vi "Get Module and FPGA Data.vi"(8 "error in (no error)":errorcluster, 11 "Parent Ref in":T2 format="%.0x") -> (0 "error out":errorcluster, 1 "RSI Modules":T10[](array[typedef]) {"Module Config Data"."Config Block Data Refs"."Data Reference" format="%.0x"; "CDOutput Data"."BD Refs"."Data Reference" format="%.0x"; "CDInput Data"."BD Refs"."Data Reference" format="%.0x"; "VS ref" format="%.0x"}, 2 "FPGA":T1[](array[typedef]) {"UDVs"."To FPGA"."VS ref" format="%.0x"; "UDVs"."From FPGA"."VS ref" format="%.0x"; "VS ref" format="%.0x"; "Output Data"."BD Refs"."Data Reference" format="%.0x"; "Input Data"."BD Refs"."Data Reference" format="%.0x"}, 3 "Parent Ref out":T2 format="%.0x", 4 "FPGALoaded":bool)   [LabVIEW 2020, in "SEECD Engine.lvlib"]
uses:
  SEECD Engine.lvlib
  <vilib>/NI VeriStand/Custom Device API/Custom Device API.lvlib
  Shared/Globals/Scan Engine GUIDs.vi
  Shared/SEECD Shared.lvlib
  <vilib>/NI VeriStand/Custom Device API/Custom Device Item Ref.ctl
  Includes/Modules.lvlibp/RSI Module/RSI Module.lvclass
  Includes/Modules.lvlibp/RSI Module/Module Models.ctl
  <vilib>/NI VeriStand/Custom Device API/Data Reference.ctl
  <vilib>/NI VeriStand/Custom Device API/Block Data Reference.ctl
  Type Defs/RSI Module Data.ctl
  Type Defs/Output Data.ctl
  Type Defs/Input Data.ctl
  Type Defs/FPGA Data.ctl
  Includes/Modules.lvlibp/RSI Module/Channel Type.ctl
  Shared/Type Defs/FXP Config.ctl
  Shared/Type Defs/UDV Data Type.ctl
  Type Defs/UDV Data.ctl
  Type Defs/Module Config Data.ctl
  Type Defs/Mixed IO.ctl
  Type Defs/Open Module IOVs.ctl
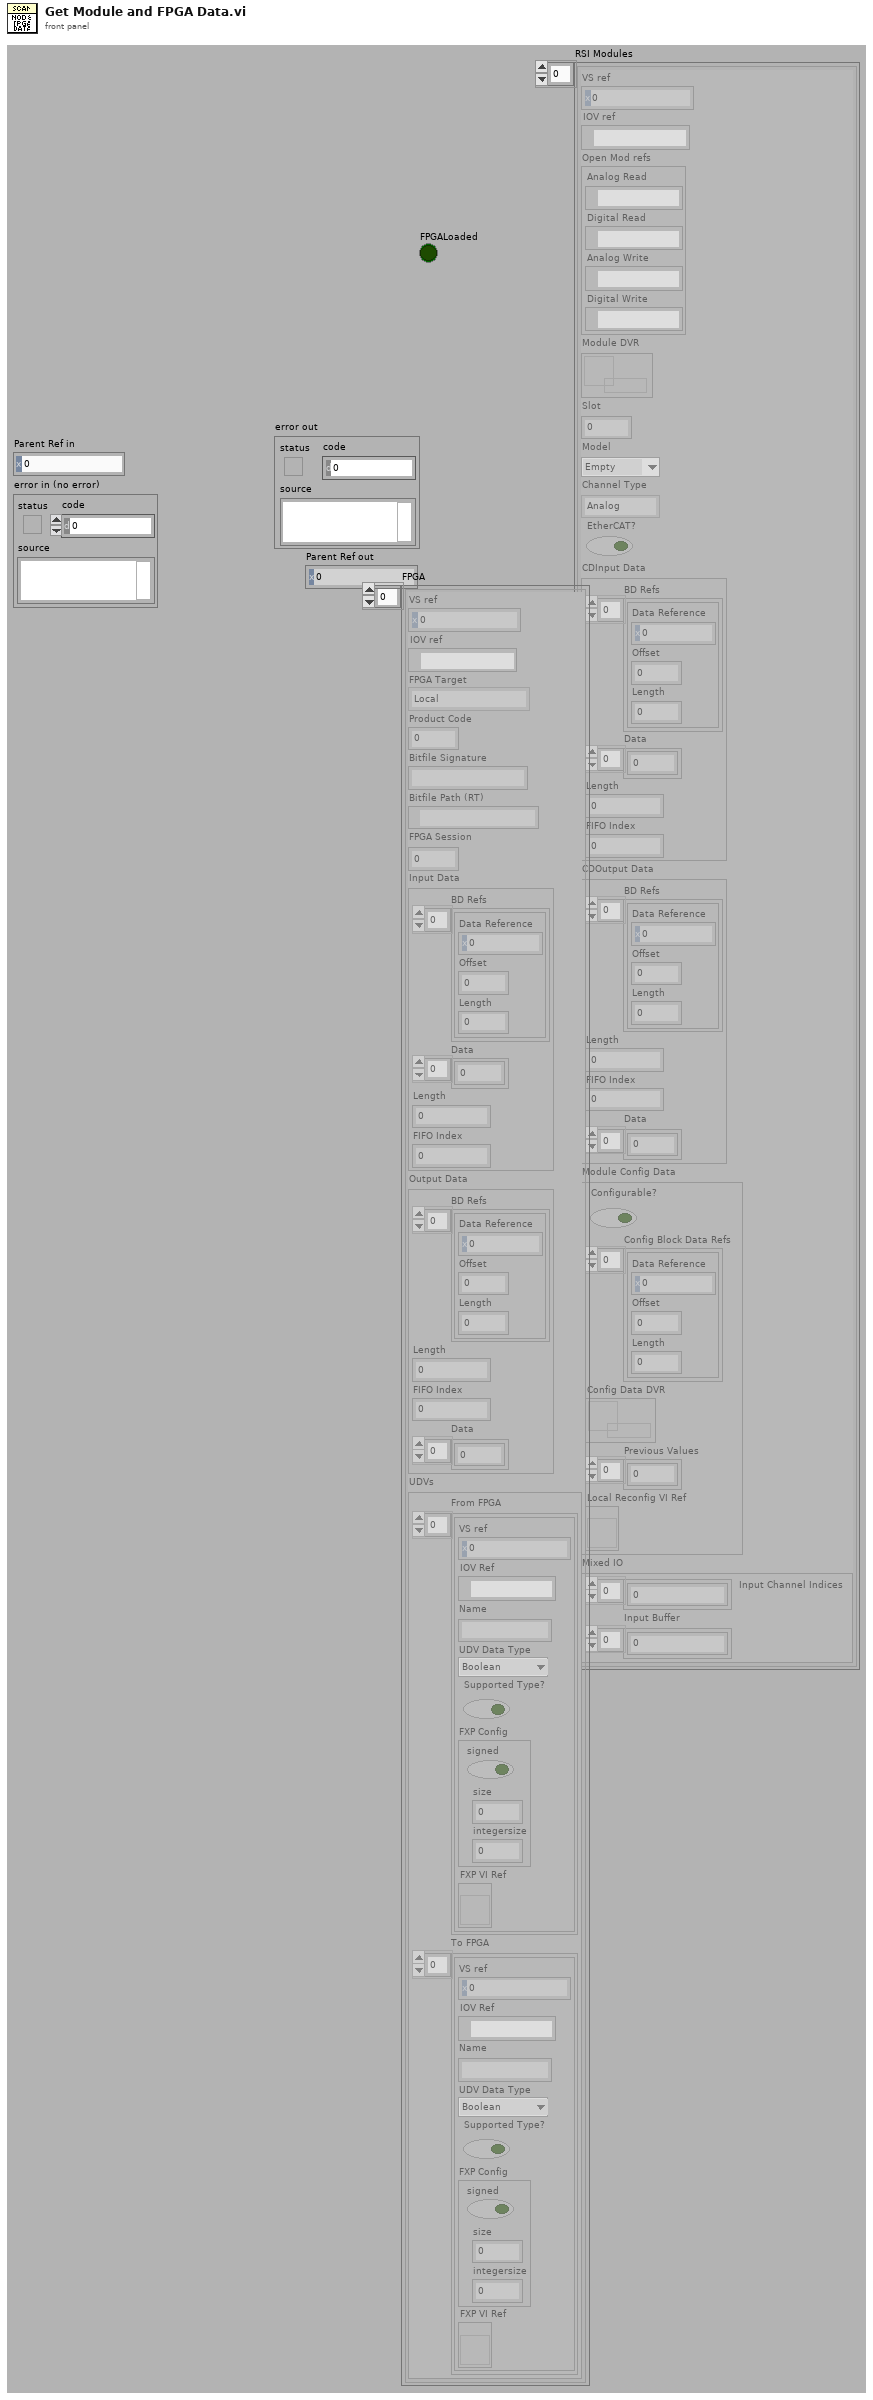
[diagram p1: front panel]
types:
  T1 = typedef "SEECD Engine.lvlib/FPGA Data.ctl" = cluster{"VS ref":T2, "IOV ref":refnum<k21>, "FPGA Target":enum16{"Local", "EtherCAT"}, "Product Code":u32, "Bitfile Signature":string, "Bitfile Path (RT)":path, "FPGA Session":u32, "Input Data":T3, "Output Data":T6, "UDVs":cluster{"From FPGA":T7[], "To FPGA":T7[]}}
  T2 = typedef "Custom Device API.lvlib/Custom Device Item Ref.ctl" = u64
  T3 = typedef "SEECD Engine.lvlib/Input Data.ctl" = cluster{"BD Refs":T4[], "Data":dbl[], "Length":i32, "FIFO Index":i32}
  T4 = typedef "Custom Device API.lvlib/Block Data Reference.ctl" = cluster{"Data Reference":T5, "Offset":u64, "Length":u64}
  T5 = typedef "Custom Device API.lvlib/Data Reference.ctl" = i32
  T6 = typedef "SEECD Engine.lvlib/Output Data.ctl" = cluster{"BD Refs":T4[], "Length":i32, "FIFO Index":i32, "Data":dbl[]}
  T7 = typedef "SEECD Engine.lvlib/UDV Data.ctl" = cluster{"VS ref":T2, "IOV Ref":refnum<k21>, "Name":string, "UDV Data Type":T8, "Supported Type?":bool, "FXP Config":T9, "FXP VI Ref":refnum<vi>}
  T8 = typedef "SEECD Shared.lvlib/UDV Data Type.ctl" = enum16{"Boolean", "Fixed Point", "Int8", "Int16", "Int32", "Int64", "U32 Bit Field", "UInt8", "UInt16", "UInt32", "UInt64", "Other", "DBL", "SGL"}
  T9 = typedef "SEECD Shared.lvlib/FXP Config.ctl" = cluster{"signed":bool, "size":u32, "integersize":i32}
  T10 = typedef "SEECD Engine.lvlib/RSI Module Data.ctl" = cluster{"VS ref":T2, "IOV ref":refnum<k21>, "Open Mod refs":T11, "Module DVR":refnum<data-value>, "Slot":u32, "Model":T12, "Channel Type":T13, "EtherCAT?":bool, "CDInput Data":T3, "CDOutput Data":T6, "Module Config Data":T14, "Mixed IO":T15}
  T11 = typedef "SEECD Engine.lvlib/Open Module IOVs.ctl" = cluster{"Analog Read":refnum<k21>, "Digital Read":refnum<k21>, "Analog Write":refnum<k21>, "Digital Write":refnum<k21>}
  T12 = typedef "Modules.lvlibp/RSI Module.lvclass/Module Models.ctl" = enum16{"Empty", "NI 9201", "NI 9203", "NI 9205", "NI 9206", "NI 9207", "NI 9208", "NI 9209", "NI 9210", "NI 9211", "NI 9212", "NI 9213", "NI 9214", "NI 9215", "NI 9216", "NI 9217", "NI 9219", "NI 9220", "NI 9221", "NI 9222", "NI 9223", "NI 9224", "NI 9225", "NI 9226", "NI 9227", "NI 9228", "NI 9229", "NI 9233", "NI 9234", "NI 9235", "NI 9236", "NI 9237", "NI 9239", "NI 9242", "NI 9244", "NI 9253", "NI 9263", "NI 9264", "NI 9265", "NI 9266", "NI 9269", "NI 9344", "NI 9350", "NI 9375", "NI 9401", "NI 9402", "NI 9403", "NI 9411", "NI 9421", "NI 9422", "NI 9423", "NI 9425", "NI 9426", "NI 9435", "NI 9436", "NI 9437", "NI 9472", "NI 9474", "NI 9475", "NI 9476", "NI 9477", "NI 9478", "NI 9481", "NI 9482", "NI 9485"}
  T13 = typedef "Modules.lvlibp/RSI Module.lvclass/Channel Type.ctl" = enum16{"Analog", "Digital"}
  T14 = typedef "SEECD Engine.lvlib/Module Config Data.ctl" = cluster{"Configurable?":bool, "Config Block Data Refs":T4[], "Config Data DVR":refnum<data-value>, "Previous Values":dbl[], "Local Reconfig VI Ref":refnum<vi>}
  T15 = typedef "SEECD Engine.lvlib/Mixed IO.ctl" = cluster{"Input Channel Indices":i32[], "Input Buffer":dbl[]}
  T16 = typedef "Modules.lvlibp/Custom Device API.lvlib/Custom Device Item Ref.ctl" = u64
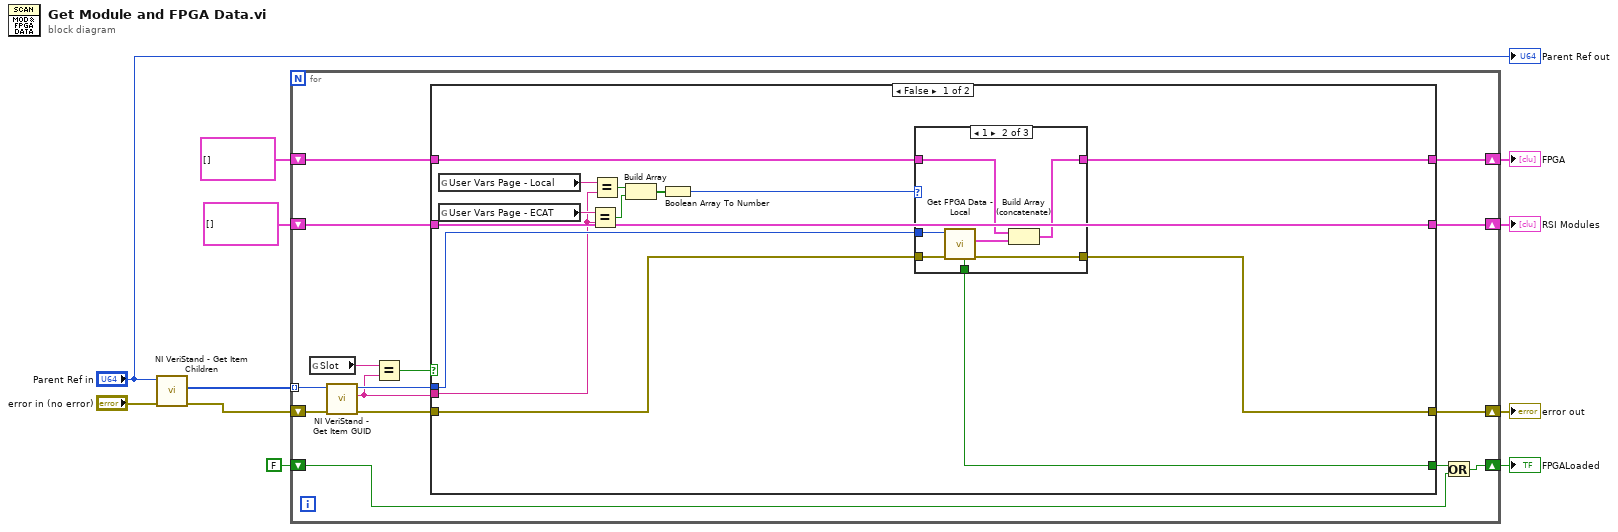
[diagram p0: block diagram]
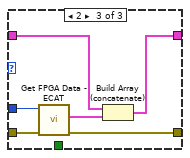
[diagram p3: hidden frame]
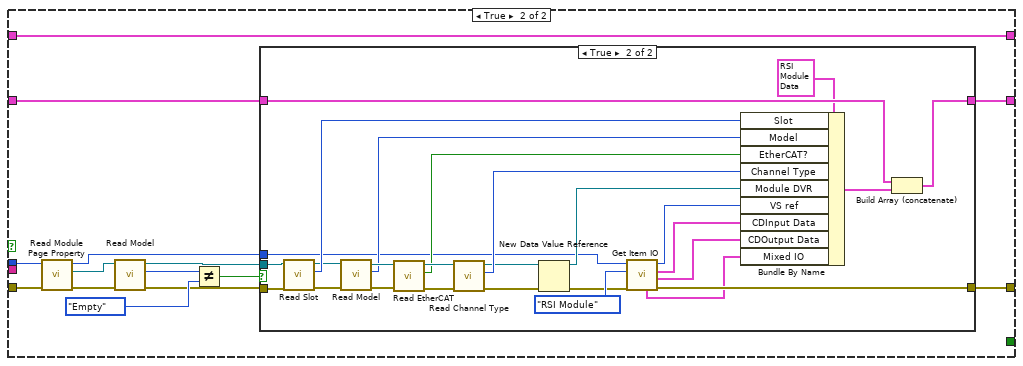
[diagram p4: hidden frame]
diagram:
  n1 = call <vilib>:"NI VeriStand - Get Item Children.vi"("error in (no error)"="error in (no error)", "Item Ref in"="Parent Ref in") -> ("error out"=w11:errorcluster, "Child Refs"=w8:T2[])  [unwired: 6 in, 2 out]
  n2 = for {
    tunnel: w8 -> [w26] mode=indexing
    shift-right: [w17] -> w5
    shift-left: w11 -> [w21]
    shift-right: [w18] -> w6
    shift-left: T10[] [] -> [w19]
    shift-right: [w15] -> w3
    shift-left: T1[] [] -> [w16]
    shift-right: [w12] -> w1
    shift-left: FALSE ("FPGALoaded") -> [w14]
    n3 = global read "Scan Engine GUIDs.vi" "Slot"() -> (w25:string)
    n4 = call <vilib>:"NI VeriStand - Get Item GUID.vi"("error in (no error)"=w21, "Item Ref in"=w26) -> ("error out"=w20:errorcluster, "GUID"=w22:string, "Item Ref out"=w24:T2)  [unwired: 7 in]
    n5 = Equal?(x=w25, y=w22) -> (x = y?=w23:bool)
    n6 = case shown="False" w23 {
      tunnel: w24 -> [w38 w62]
      tunnel: w22 -> [w32 _]
      tunnel: w20 -> [w37 w63]
      tunnel: w19 -> [w40 w67]
      tunnel: [w40 w66] -> w18
      tunnel: [w36 w65] -> w17
      tunnel: w16 -> [w39 w64]
      tunnel: [w35 w64] -> w15
      tunnel: [w27 _] -> w13
      frame False {
        n7 = global read "Scan Engine GUIDs.vi" "User Vars Page - Local"() -> (w34:string)
        n8 = global read "Scan Engine GUIDs.vi" "User Vars Page - ECAT"() -> (w33:string)
        n9 = Equal?(x=w33, y=w32) -> (x = y?=w29:bool)
        n10 = Equal?(x=w34, y=w32) -> (x = y?=w30:bool)
        n11 = Build Array(w30, w29) -> (w31:bool[])
        n12 = Boolean Array To Number(Boolean array=w31) -> (number=w28:u32)
        n13 = case shown="1" w28 {
          tunnel: w39 -> [w41 w48 w55]
          tunnel: w38 -> [_ w47 w53]
          tunnel: w37 -> [w42 w46 w52]
          tunnel: [w42 w44 w50] -> w36
          tunnel: [w41 w49 w54] -> w35
          tunnel: [_ w43 _] -> w27
          frame 0, Default {
          }
          frame 1 {
            n14 = call "Get FPGA Data - Local.vi"("error in (no error)"=w46, "Item Ref in"=w47) -> ("error out"=w44:errorcluster, "FPGA"=w45:T1, "FPGALoaded"=w43:bool)  [unwired: 6 in, 1 out]
            n15 = Build Array (concatenate)(w48, w45) -> (w49:T1[])
          }
          frame 2 {
            n16 = call "Get FPGA Data - ECAT.vi"("error in (no error)"=w52, "Item Ref in"=w53) -> ("error out"=w50:errorcluster, "FPGA"=w51:T1)  [unwired: 7 in, 1 out]
            n17 = Build Array (concatenate)(w55, w51) -> (w54:T1[])
          }
        }
      }
      frame True {
        n18 = call "Read Module Page Property.vi"("error in (no error)"=w63, "Node Ptr In"=w62) -> ("error out"=w61:errorcluster, "RSI Module"=w58:refnum<class "RSI Module.lvclass">, "Node Ptr Out"=w57:T16)  [unwired: 7 in]
        n19 = call "Read Model.vi"("error in (no error)"=w61, "RSI Module in"=w58) -> ("error out"=w59:errorcluster, "Model"=w60:T12, "RSI Module out"=w56:refnum<class "RSI Module.lvclass">)  [unwired: 7 in]
        n20 = Not Equal?(x=w60, y=Module_Models."Empty" ("x")) -> (x != y?=w68:bool)
        n21 = case shown="True" w68 {
          tunnel: w67 -> [w71 w98]
          tunnel: [w71 w97] -> w66
          tunnel: [w70 w77] -> w65
          tunnel: w59 -> [w70 w86]
          tunnel: w57 -> [_ w74]
          tunnel: w56 -> [_ w87]
          frame False {
          }
          frame True {
            n22 = call "Read Slot.vi"("error in (no error)"=w86, "RSI Module in"=w87) -> ("error out"=w83:errorcluster, "Slot"=w85:u32, "RSI Module out"=w84:refnum<class "RSI Module.lvclass">)  [unwired: 7 in]
            n23 = call "Read Model.vi"("error in (no error)"=w83, "RSI Module in"=w84) -> ("error out"=w82:errorcluster, "Model"=w80:T12, "RSI Module out"=w81:refnum<class "RSI Module.lvclass">)  [unwired: 7 in]
            n24 = call "Read EtherCAT.vi"("error in (no error)"=w82, "RSI Module in"=w81) -> ("error out"=w90:errorcluster, "EtherCAT?"=w89:bool, "RSI Module out"=w91:refnum<class "RSI Module.lvclass">)  [unwired: 7 in]
            n25 = call "Read Channel Type.vi"("error in (no error)"=w90, "RSI Module in"=w91) -> ("error out"=w76:errorcluster, "Channel Type"=w92:T13, "RSI Module out"=w75:refnum<class "RSI Module.lvclass">)  [unwired: 7 in]
            n26 = New Data Value Reference(data value=w75, error in=w76) -> (data value reference=w78:refnum<data-value>, error out=w88:errorcluster)
            n27 = call "Get Item IO.vi"("error in (no error)"=w88, "Item Type"=enum16{"RSI Module", "User Variables"}."RSI Module", "Item Ref in"=w74) -> ("error out"=w77:errorcluster, "Output Data"=w94:T6, "Input Data"=w95:T3, "Item Ref out"=w79:T2, "Mixed IO"=w73:T15)  [unwired: 2 in, 2 out]
            n28 = Bundle By Name(cluster=T10 {"VS ref"=0, "IOV ref"="", "Open Mod refs"={"Analog Read"="", "Digital Read"="", "Analog Write"="", "Digital Write"=""}, "Module DVR"=refnum, "Slot"=0, "Model"=enum."Empty", "Channel Type"=enum."Analog", "EtherCAT?"=FALSE, "CDInput Data"={"BD Refs"=[], "Data"=[], "Length"=0, "FIFO Index"=0}, "CDOutput Data"={"BD Refs"=[], "Length"=0, "FIFO Index"=0, "Data"=[]}, "Module Config Data"={"Configurable?"=FALSE, "Config Block Data Refs"=[], "Config Data DVR"=refnum, "Previous Values"=[], "Local Reconfig VI Ref"=refnum}, "Mixed IO"={"Input Channel Indices"=[], "Input Buffer"=[]}} ("RSI Module"), "Slot"=w85, "Model"=w80, "EtherCAT?"=w89, "Channel Type"=w92, "Module DVR"=w78, "VS ref"=w79, "CDInput Data"=w95, "CDOutput Data"=w94, "Mixed IO"=w73) -> (w96:T10)
            n29 = Build Array (concatenate)(w98, w96) -> (w97:T10[])
          }
        }
      }
    }
    n30 = Or(x=w13, y=w14) -> (x .or. y?=w12:bool)
  }
  "RSI Modules" <- w6
  "error out" <- w5
  "FPGA" <- w3
  "FPGALoaded" <- w1
  "Parent Ref out" <- "Parent Ref in"
